vi "host.vi"() -> ()   [LabVIEW 2018]
uses:
  <vilib>/userdefined/High Color/nirio_resource_hc.ctl
  <instrlib>/niDCPower/nidcpower.llb/niDCPower Measurement Type.ctl
  <vilib>/FPGAPlugInAG/PXI-7953R/niLvFpga_Open_PXI-7953R.vi
  <vilib>/rvi/interface/common/dynamic/niFpgaDynamicAddResources.vi
  <vilib>/FPGAPlugInAG/Dynamic/niLvFpga_Reset_Dynamic.vi
  <vilib>/FPGAPlugInAG/Dynamic/niLvFpga_Run_Dynamic.vi
  <vilib>/Utility/error.llb/Error Cluster From Error Code.vi
  <vilib>/rvi/errors/niLvFpgaAdjustHostInterfaceError.vi
  <vilib>/FPGAPlugInAG/Dynamic/niLvFpga_Close_Dynamic.vi
  <vilib>/rvi/interface/nirviOpenFPGA/nirviOpenFPGA.xnode
  FPGA Bitfiles/matrix_FPGATarget_Matrixtarget_8M6uhoGy8lc.lvbitx
  <vilib>/rvi/interface/nirviMethod/nirviMethod.xnode
  <vilib>/rvi/interface/nirviReadWriteControl/nirviReadWriteControl.xnode
  <vilib>/rvi/interface/nirviCloseFPGA/nirviCloseFPGA.xnode
  <vilib>/FPGAPlugInAG/Dynamic/niLvFpga_ReadFifo_Dynamic.vi
  <vilib>/rvi/errors/niLvFpgaMergeErrorWithErrorCode.vi
  <vilib>/rvi/interface/Simulation/niFpgaSimulationCallBeginRW.vi
  <vilib>/vision/NI_Vision_Development_Module.lvlib
  NiFpgaLv.dll
panel:
  in  "57":i16=57
  in  "91":i16=91
  in  "Index - Registers Page 1":u16[](array[numeric])=[5, 6, 8, 16, 17, 18, 27, 28, 30, 37, 52, 53, 58, 59, 60, 71, 72, 76, 77, 78, 82, 83, 84, 85, 86, 87, 88, 104, 128, 129, 130, 131, 132, 133, 134, 135, 136, 137, 138, 139, 140, 141, 142, 143, 144, 145, 146, 147, 148, 149, 155, 157, 159, 160, 161, 162, 163, 164, 165, 166, 167, 168, 169, 170, 174, 175, 179, 180, 181, 182, 183, 184, 185, 186, 187, 188, 189, 190, 191, 192, 193, 194, 195, 196, 200, 220, 221, 222, 223, 224, 225, 226, 227, 240]
  in  "Registers Page 1":u16[](array[numeric])=[3, 28686, 128, 61437, 64831, 16367, 0, 0, 512, 5, 16, 61456, 512, 1066, 1024, 24, 0, 0, 0, 10, 0, 7700, 17966, 34666, 47008, 57548, 0, 17, 7, 56588, 62696, 1276, 57868, 63212, 764, 56588, 62696, 250, 34866, 56754, 63466, 2, 47646, 60627, 63473, 255, 48926, 61142, 63474, 3, 512, 9390, 0, 1280, 1280, 0, 1024, 1024, 0, 1280, 640, 0, 1024, 512, 1284, 16, 2, 32, 257, 4363, 15399, 4362, 12834, 5643, 12836, 9228, 24124, 127, 8200, 20023, 100, 8463, 19250, 100, 0, 7700, 17966, 34666, 47008, 57548, 0, 28672, 45091, 0] format="%x"
  out "Glitch Registers 2":string
  out "Glitch Registers":string
  out "glitch_num":i32
  out "Data_Read":u16=65535 format="%x"
  in  "Index - Registers Page 0":u16[](array[numeric])=[0, 1, 2, 3, 4, 5, 6, 7, 8, 9, 10, 11, 12, 13, 31, 32, 33, 34, 35, 36, 43, 44, 45, 46, 47, 48, 49, 50, 51, 52, 54, 55, 59, 60, 61, 62, 63, 64, 65, 66, 89, 90, 95, 96, 97, 98, 99, 100, 101, 112, 113, 114, 115, 116, 117, 118, 119, 120, 121, 122, 123, 124, 125, 126, 128, 129, 130, 131, 132, 133, 134, 135, 200, 240, 245, 246, 247, 248, 249, 250, 251, 252, 253, 255, 0]
  in  "Registers Page 0":u16[](array[numeric])=[5178, 12, 30, 1024, 1280, 388, 42, 190, 17, 537, 17, 0, 0, 8, 0, 768, 1036, 297, 1544, 32875, 32, 32, 32, 32, 32, 1066, 7168, 0, 841, 49177, 61680, 0, 33, 6688, 8222, 8224, 8224, 8220, 215, 1911, 12, 49167, 8989, 128, 0, 0, 0, 0, 0, 31498, 31498, 6414, 6159, 22322, 22068, 29493, 12306, 30978, 29958, 30474, 30729, 32006, 12560, 126, 127, 127, 22282, 22539, 18188, 18446, 23298, 92, 0, 0, 2047, 2047, 0, 0, 124, 0, 0, 0, 0, 5178] format="%x"
  out "number":u64=18446744073709551615 format="%b"
  in  "WRITE\nSEL_LOG":bool=TRUE caption="SEL LOGS"
  out "SEL_log file":refnum<file>
  out "IS_SEL":bool
  in  "SIM_SEL":bool
  in  "VDDIO_limit, mA":dbl=500.0 format="%#_13g"
  in  "VAA_limit, mA":dbl=500.0 format="%#_13g"
  out "selNumVAA":i32 caption="selNum"
  out "selNumVDDIO":i32 caption="selNum"
  in  "voltage level VAA":dbl=2.8 format="%#_13g"
  in  "voltage level VDD":dbl=2.8 format="%#_13g"
  in  "current limit VAA":dbl=0.10000000000000009 format="%#_13g"
  in  "current limit VDD":dbl=0.09999999999999995 format="%#_13g"
  in  "SEL":path=path "C:/VPL/LabView_PRJ/ПЕЛЕНГ_CMV4000/LOGS/SEL"
  out "Температура":string="0"
  out "Номер образца":string="0"
  out "VDDIO_Current, mA":dbl=1.2009055104110689 caption="mA" format="%_5g"
  out "VDDIO_Voltage, V":dbl=2.8003152785592405 caption="V" format="%_4g"
  out "VAA_Current, mA":dbl=14.742607861326585 caption="mA" format="%_5g"
  out "VAA_Voltage, V":dbl=2.799911738250357 caption="V" format="%_4g"
  in  "VAA - VAAPIX":refnum<k15>="PXI1Slot3"
  in  "SEL_time":u32=100
  out "Read_Low":u8=255 format="%x"
  out "Read_Up":u8=255 format="%x"
  out "TIRISTOR":bool
  in  "/RESET":bool=TRUE
  in  "DataLow":u8=231 format="%x"
  in  "Reg":u8=244 format="%x"
  in  "DataUp":u8=2 format="%x"
  in  "Device":u8=186 format="%x"
  in  "VDD_limit, mA":dbl=500.0 format="%#_13g"
  out "selNumVDD":i32 caption="selNum"
  out "Ready":bool=TRUE
  in  "output enabled":bool=TRUE
  out "VDD_Current, mA":dbl=-0.2678676595787411 caption="mA" format="%_5g"
  out "VDD_Voltage, V":dbl=2.801952990328096 caption="V" format="%_4g"
  in  "VDDIO - VDD":refnum<k15>="PXI1Slot2"
  in  "Comand":T1(ring)=enum."From Controls"
  in  "Height_pix":i32=250
  in  "Width_pix":i32=250
  in  "55":i16=55
  in  "73":i16=73
  in  "75":i16=75
  in  "56":i16=56
  in  "55":i16=55
  in  "Comand":bool
  out "ACK":u8 format="%b"
  out "String_counter":i16=250
  in  "String_number":i16=250
  in  "I2C_Request":bool
  in  "FALSE_LV":bool
  in  "FALSE_PIXCLK":bool=TRUE
  in  "TRUE_FV":bool=TRUE
  in  "1_EXTCLK_divider":i16=5
  out "Image":T2(plugin-control)
  in  "0_WE divider":i32
  in  "50_Rise/Fall divider":i32=50
  in  "72":i16=72
  in  "18":i16=18
  in  "36":i16=36
  in  "54":i16=54
  in  "71":i16=71
  in  "17":i16=17
  in  "35":i16=35
  in  "53":i16=53
  in  "75_Stop":i16=75
  in  "100_Sclk_divider":i32=100
  in  "Read1":u8=255 format="%x"
  in  "Read2":u8=255 format="%x"
  in  "I2C_Write":bool
  in  "stop":bool=TRUE
  out "ArrayUp":u64=1534
  out "ArrayLow":u64=2298524764643157990
  in  "resource name":T3="PXI1Slot6" caption="RIO Device"
  out "Сколько вначале":u32=262142
  out "Data":u8[](array[numeric])
  # "YCbCr mode"
  # "VDD"
  # "VDDIO"
  # "VAA"
  # "RGB565"
  # "I2C"
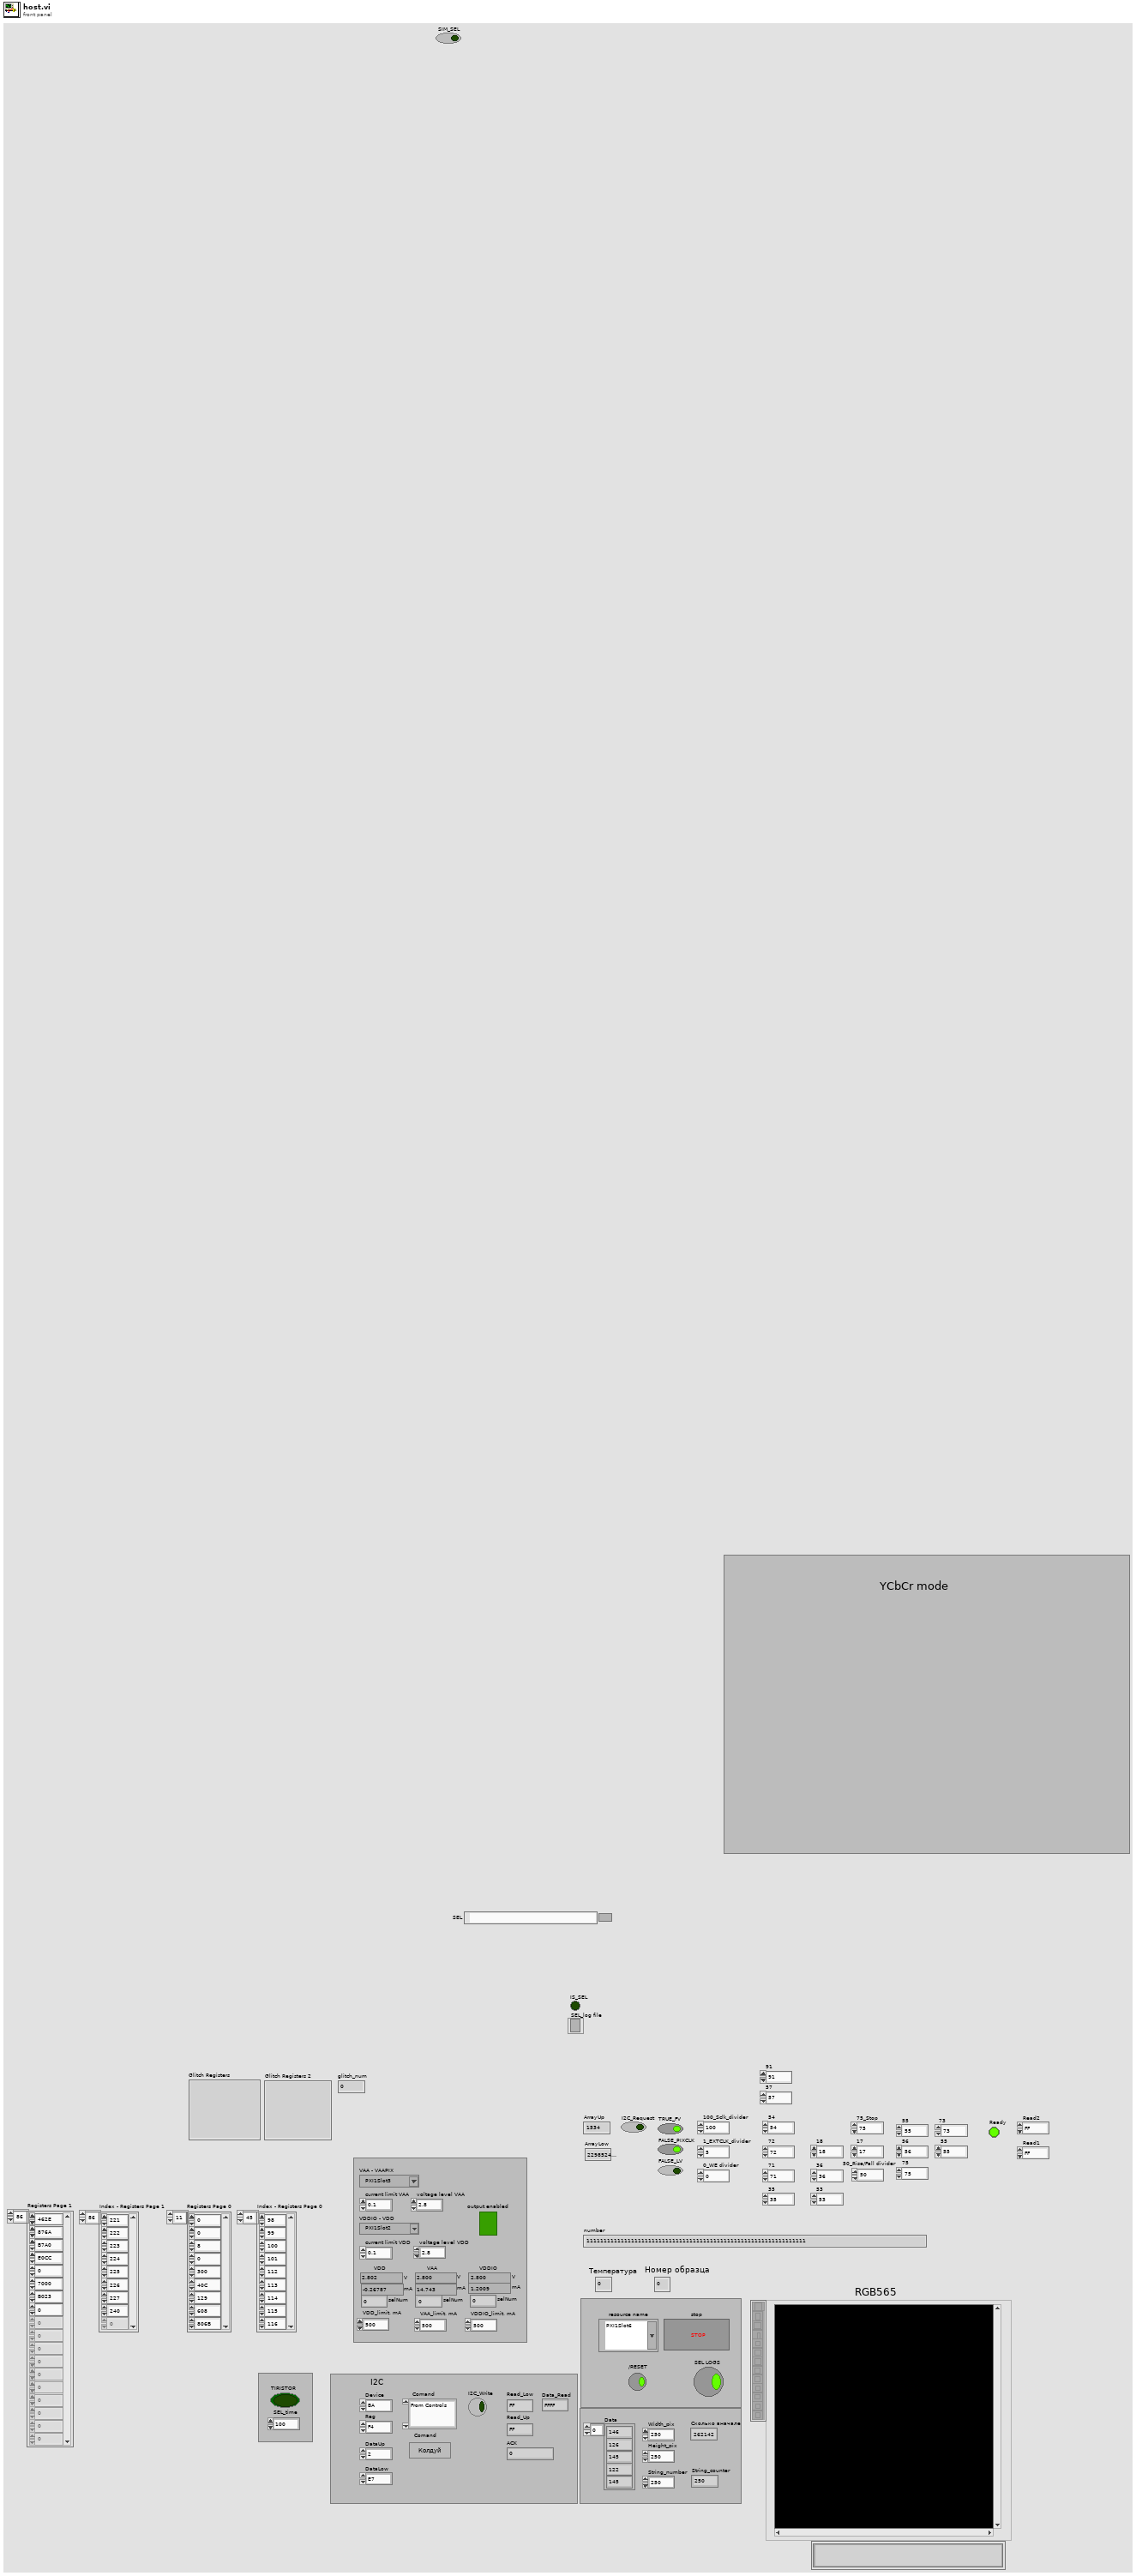
[diagram p1: front panel]
types:
  T1 = enum16{"check_registers", "From Controls", "250x250", "RGB565"}
  T2 = typedef "IMAQ Image.ctl" = refnum<image>
  T3 = typedef "nirio_resource_hc.ctl" = tag
  T4 = enum16{"open", "replace", "create", "open or create", "replace or create", "replace or create with confirmation"}
  T5 = typedef "Image Type" = u32
  T6 = typedef "niDCPower Measurement Type.ctl" = i32
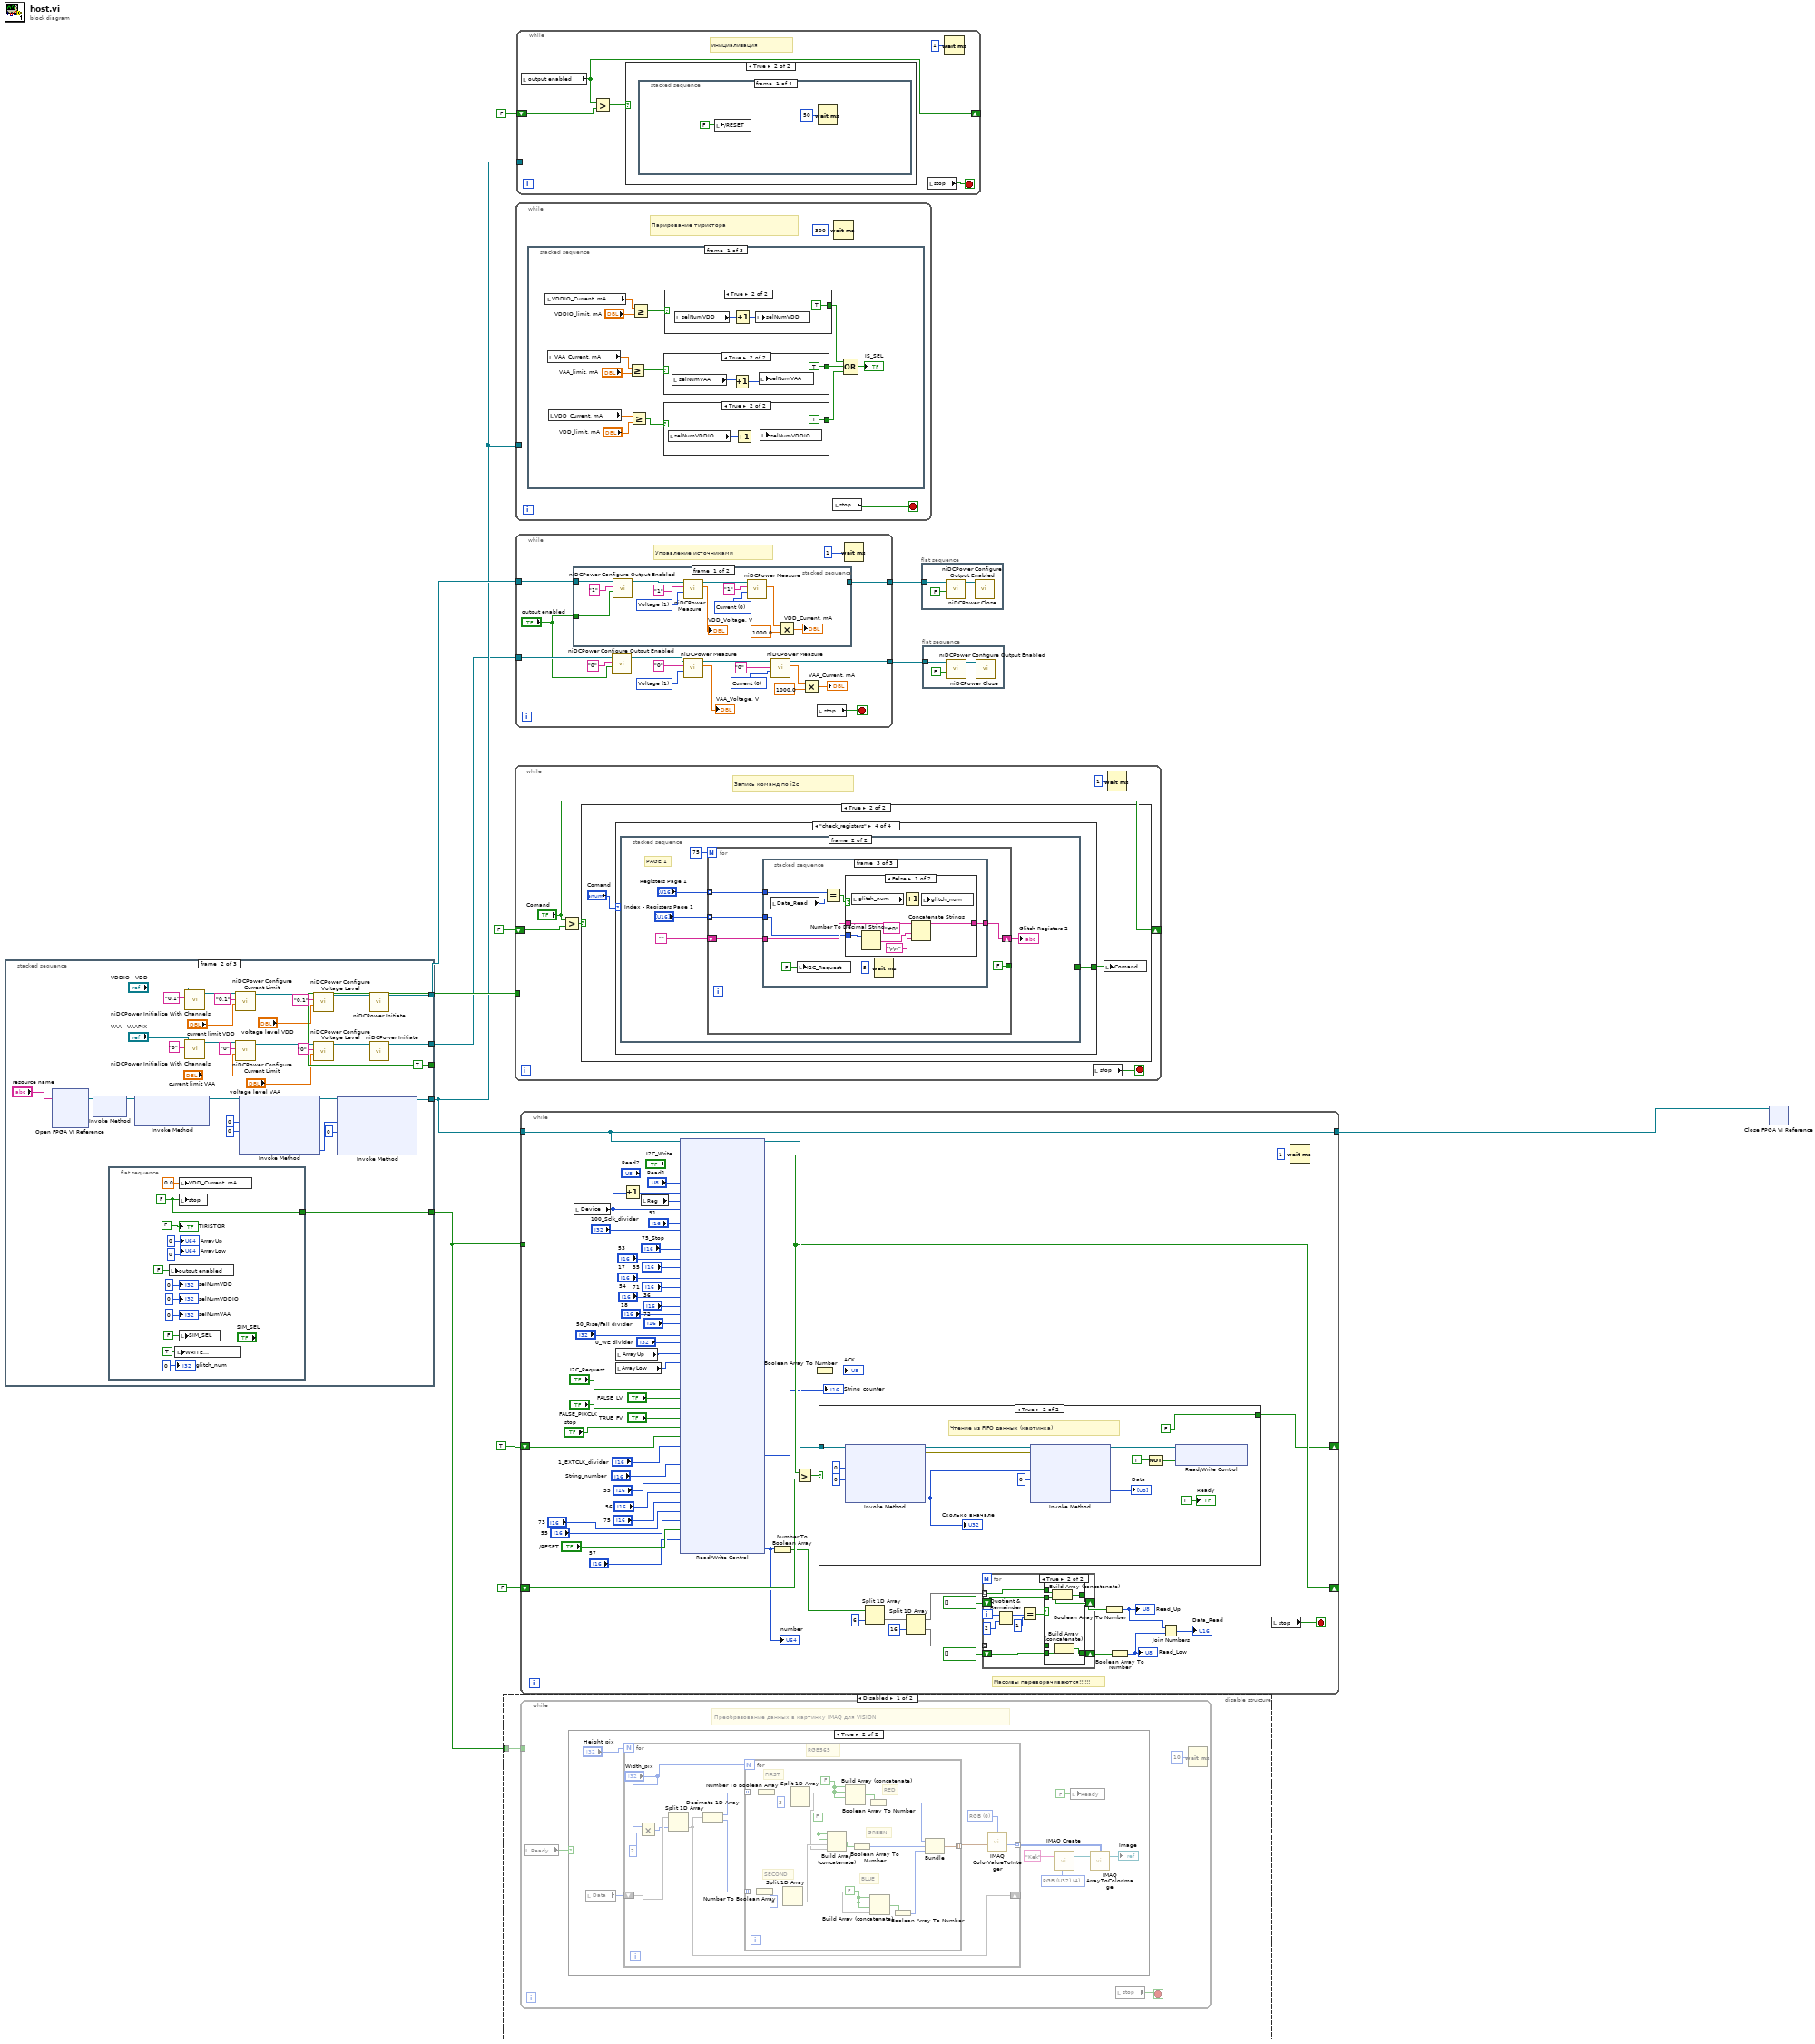
[diagram p0: block diagram]
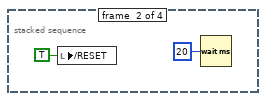
[diagram p5: hidden frame]
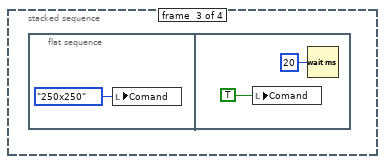
[diagram p6: hidden frame]
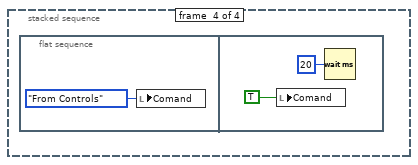
[diagram p7: hidden frame]
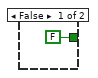
[diagram p8: hidden frame]
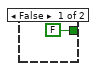
[diagram p9: hidden frame]
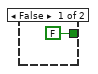
[diagram p10: hidden frame]
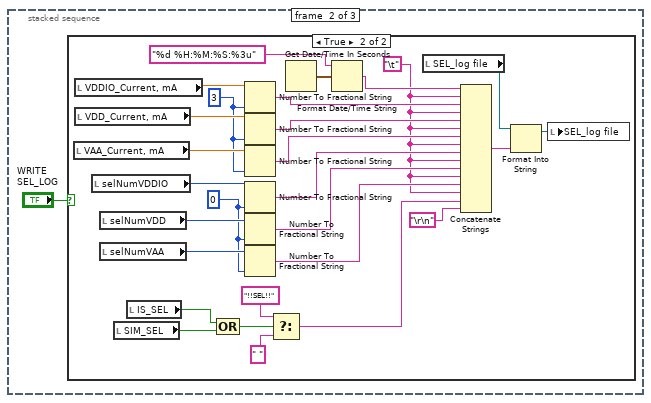
[diagram p11: hidden frame]
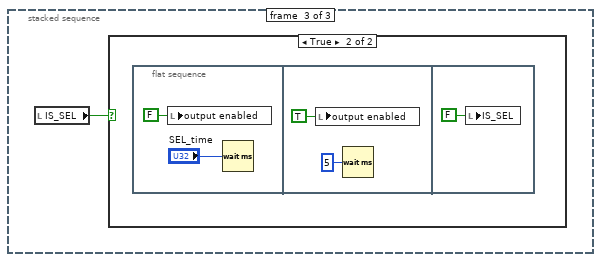
[diagram p13: hidden frame]
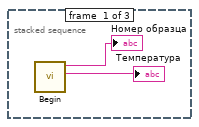
[diagram p15: hidden frame]
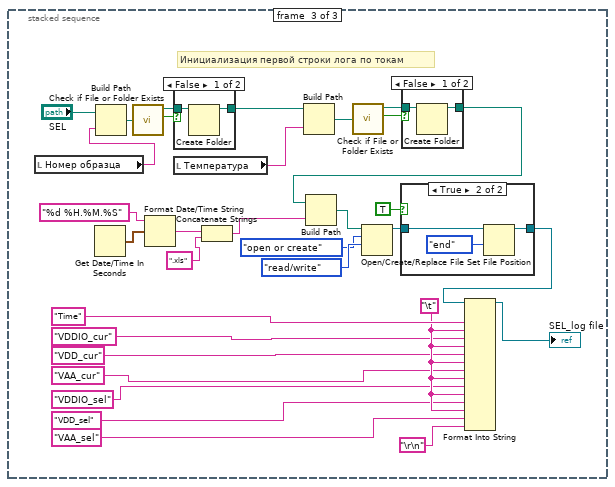
[diagram p16: hidden frame]
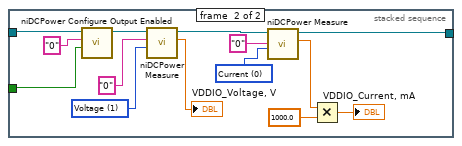
[diagram p20: hidden frame]
diagram:
  n1 = stacked-sequence {
    tunnel: [_ w46 _] -> w3
    tunnel: [_ w27 _] -> w5
    tunnel: [_ w26 _] -> w7
    tunnel: [_ TRUE _] -> w6
    tunnel: [_ w15 _] -> w2
    frame #0 {
      n2 = call "Begin.vi"() -> ("Температура 2"=→"Температура":string, "Номер образца 2"=→"Номер образца":string)  [unwired: 10 in]
    }
    frame #1 {
      n3 = xnode "Open FPGA VI Reference"("resource name"="resource name") -> ("FPGA VI Reference Out"=w36:refnum<k20>)  [unwired: 1 in, 1 out]
      n4 = xnode "Invoke Method"("FPGA VI Reference In"=w36) -> ("FPGA VI Reference Out"=w35:refnum<k20>)  [unwired: 1 in, 1 out]
      n5 = flat-sequence {
        tunnel: [w58] -> w27
        frame #0 {
          w58 = FALSE ("СТОП ПЛИС")
          n6 = local write "output enabled"(FALSE ("output enabled")) -> ()
          n7 = local write "WRITE\nSEL_LOG"(TRUE ("WRITE\nSEL_LOG")) -> ()
          n8 = local write "VDD_Current, mA"(0.0 ("Ch1_Current, mA")) -> ()
          n9 = local write "stop"(w58) -> ()
          n10 = local write "SIM_SEL"(FALSE ("SIM_SEL")) -> ()
          "ArrayLow" <- u64 0 ("ArrayLow")
          "ArrayUp" <- u64 0 ("ArrayUp")
          "selNumVDD" <- 0 ("Numeric")
          "TIRISTOR" <- FALSE ("TIRISTOR")
          "selNumVDDIO" <- 0 ("Numeric")
          "selNumVAA" <- 0 ("Numeric")
          "glitch_num" <- 0 ("glitch_num")
        }
      }
      n11 = xnode "Invoke Method"("FPGA VI Reference In"=w35) -> ("FPGA VI Reference Out"=w33:refnum<k20>)  [unwired: 2 in, 1 out]
      n12 = call <instrlib>:"niDCPower Initialize With Channels.vi"("channels"="0,1", "resource name"="VDDIO - VDD") -> ("instrument handle out"=w37:refnum<k15>)  [unwired: 8 in, 1 out]
      n13 = call <instrlib>:"niDCPower Initialize With Channels.vi"("channels"="0", "resource name"="VAA - VAAPIX") -> ("instrument handle out"=w16:refnum<k15>)  [unwired: 8 in, 1 out]
      n14 = call <instrlib>:"niDCPower Configure Current Limit.vi"("current limit"="current limit VDD", "channel name"="0,1", "instrument handle"=w37) -> ("instrument handle out"=w38:refnum<k15>)  [unwired: 7 in, 1 out]
      n15 = call <instrlib>:"niDCPower Configure Current Limit.vi"("current limit"="current limit VAA", "channel name"="0", "instrument handle"=w16) -> ("instrument handle out"=w17:refnum<k15>)  [unwired: 7 in, 1 out]
      n16 = xnode "Invoke Method"("FPGA VI Reference In"=w33, "Number of Elements"=u32 0, "Timeout (ms)"=0) -> ("FPGA VI Reference Out"=w31:refnum<k20>, "Elements Remaining"=w32:u32)  [unwired: 1 in, 2 out]
      n17 = call <instrlib>:"niDCPower Configure Voltage Level.vi"("voltage level"="voltage level VDD", "channel name"="0,1", "instrument handle"=w38) -> ("instrument handle out"=w39:refnum<k15>)  [unwired: 7 in, 1 out]
      n18 = call <instrlib>:"niDCPower Configure Voltage Level.vi"("voltage level"="voltage level VAA", "channel name"="0", "instrument handle"=w17) -> ("instrument handle out"=w18:refnum<k15>)  [unwired: 7 in, 1 out]
      n19 = xnode "Invoke Method"("FPGA VI Reference In"=w31, "Number of Elements"=w32, "Timeout (ms)"=0) -> ("FPGA VI Reference Out"=w46:refnum<k20>)  [unwired: 1 in, 3 out]
      n20 = call <instrlib>:"niDCPower Initiate.vi"("instrument handle"=w39) -> ("instrument handle out"=w26:refnum<k15>)  [unwired: 9 in, 1 out]
      n21 = call <instrlib>:"niDCPower Initiate.vi"("instrument handle"=w18) -> ("instrument handle out"=w15:refnum<k15>)  [unwired: 9 in, 1 out]
    }
    frame #2 {
      w67 = "\t"
      # "Инициализация первой строки лога по токам"
      n22 = local read "Номер образца"() -> (w78:string)
      n23 = Get Date/Time In Seconds() -> (seconds since 1Jan1904=w83:timestamp)
      n24 = Build Path(base path="SEL", name or relative path=w78) -> (appended path=w76:path)
      n25 = call <vilib>:"Check if File or Folder Exists.vi"("path"=w76) -> ("file or folder exists?"=w75:bool, "dup path"=w74:path)  [unwired: 8 in, 1 out]
      n26 = Format Date/Time String(time format string (%c)="%d %H.%M.%S", seconds (now)=w83) -> (date/time string=w85:string)  [unwired: 1 in]
      n27 = case shown="False" w75 {
        tunnel: w74 -> [w99 w100]
        tunnel: [w98 w100] -> w80
        frame False {
          n28 = Create Folder(path (use dialog)=w99) -> (created path=w98:path)  [unwired: 2 in, 2 out]
        }
        frame True {
        }
      }
      n29 = local read "Температура"() -> (w81:string)
      n30 = Concatenate Strings(w85, ".xls" ("string")) -> (w86:string)
      n31 = Build Path(base path=w80, name or relative path=w81) -> (appended path=w89:path)
      n32 = call <vilib>:"Check if File or Folder Exists.vi"("path"=w89) -> ("file or folder exists?"=w90:bool, "dup path"=w79:path)  [unwired: 8 in, 1 out]
      n33 = case shown="False" w90 {
        tunnel: w79 -> [w96 w97]
        tunnel: [w95 w97] -> w87
        frame False {
          n34 = Create Folder(path (use dialog)=w96) -> (created path=w95:path)  [unwired: 2 in, 2 out]
        }
        frame True {
        }
      }
      n35 = Build Path(base path=w87, name or relative path=w86) -> (appended path=w84:path)
      n36 = Open/Create/Replace File(file path (use dialog)=w84, operation (0:open)=T4."open or create", access (0:read/write)=enum16{"read/write", "read-only", "write-only"}."read/write") -> (refnum out=w82:refnum<file>)  [unwired: 3 in, 2 out]
      n37 = case shown="True" TRUE {
        tunnel: w82 -> [w91 w94]
        tunnel: [w91 w92] -> w88
        frame False {
        }
        frame True {
          n38 = Set File Position(refnum=w94, from (0:start)=enum16{"start", "end", "current"}."end") -> (refnum out=w92:refnum<file>)  [unwired: 2 in, 1 out]
        }
      }
      n39 = Format Into String(initial string=w88, "Time" ("input 1"), w67, "VDDIO_cur" ("input 1"), w67, "VDD_cur" ("input 1"), w67, "VAA_cur" ("input 1"), w67, "VDDIO_sel" ("input 1"), w67, "VDD_sel" ("input 1"), w67, "VAA_sel" ("input 1"), "\r\n") -> (resulting string=→"SEL_log file":refnum<file>)  [unwired: 2 in, 1 out]
    }
  }
  n40 = disable-structure shown="Disabled" {
    disable-tunnel: w5 -> [w101 _]
    frame Disabled {
      n41 = while {
        tunnel: w101 -> [_]
        stop <- w104 stop-if-true
        # "Преобразование данных в картинку IMAQ для VISION"
        n42 = local read "Ready"() -> (w102:bool)
        n43 = case shown="True" w102 {
          frame False {
          }
          frame True {
            w111 = T5 4 items=["Grayscale (U8)", "Grayscale (I16)", "Grayscale (SGL)", "Complex (CSG)", "RGB (U32)", "HSL (U32)", "RGB (U64)"] ("Image Type")
            n44 = local read "Data"() -> (w106:u8[])
            n45 = for {
              N: "Height_pix" -> [_]
              shift-right: [w118] -> _
              shift-left: w106 -> [w115]
              tunnel: [w116] -> w107 mode=indexing
              w120 = u16 0 items=["RGB", "HSL", "HSV", "HSI"] ("Color Mode")
              # "RGB565"
              n46 = Multiply(x="Width_pix", y=2) -> (x*y=w114:i32)
              n47 = Split 1D Array(array=w115, index=w114) -> (second subarray=w118:u8[])  [unwired: 1 out]
              n48 = Decimate 1D Array(w118) -> (w122:u8[], w121:u8[])
              n49 = for {
                N: "Width_pix" -> [_]
                tunnel: w122 -> [w141] mode=indexing
                tunnel: w121 -> [w142] mode=indexing
                tunnel: [w123] -> w117 mode=indexing
                w131 = FALSE
                w132 = FALSE
                w133 = FALSE
                # "BLUE"
                # "GREEN"
                # "RED"
                # "SECOND"
                # "FIRST"
                n50 = Number To Boolean Array(number=w142) -> (Boolean array=w137:bool[])
                n51 = Number To Boolean Array(number=w141) -> (Boolean array=w140:bool[])
                n52 = Split 1D Array(array=w137, index=5) -> (first subarray=w129:bool[], second subarray=w136:bool[])
                n53 = Split 1D Array(array=w140, index=3) -> (first subarray=w128:bool[], second subarray=w127:bool[])
                n54 = Build Array (concatenate)(w132, w132, w136, w128) -> (w135:bool[])
                n55 = Build Array (concatenate)(w133, w133, w133, w127) -> (w134:bool[])
                n56 = Boolean Array To Number(Boolean array=w135) -> (number=w125:u8)
                n57 = Boolean Array To Number(Boolean array=w134) -> (number=w124:u8)
                n58 = Build Array (concatenate)(w131, w131, w131, w129) -> (w130:bool[])
                n59 = Boolean Array To Number(Boolean array=w130) -> (number=w126:u8)
                n60 = Bundle(w124, w125, w126) -> (w123:cluster{u8, u8, u8})  [unwired: 1 in]
              }
              n61 = call "IMAQ ColorValueToInteger"("1D Color value array"=w117, "Color Mode"=w120) -> ("1D U32 array"=w116:u32[])  [unwired: 3 in, 3 out]
            }
            n62 = call "IMAQ Create"("Image Name"="Kek", "Image Type"=w111) -> ("New Image"=w110:T2)  [unwired: 3 in, 1 out]
            n63 = local write "Ready"(FALSE ("Ready")) -> ()
            n64 = call "IMAQ ArrayToColorImage"("Image Pixels (U32)"=w107, "Image"=w110) -> ("Image Out"=→"Image":T2)  [unwired: 3 in, 1 out]
          }
        }
        n65 = local read "stop"() -> (w104:bool)
        n66 = Wait (ms)(milliseconds to wait=u32 10) -> ()  [unwired: 1 out]
      }
    }
    frame Enabled {
    }
  }
  n67 = while {
    shift-right: ["Comand"] -> _
    shift-left: FALSE -> [w145]
    tunnel: w6 -> [_]
    stop <- w147 stop-if-true
    # "Запись команд по i2c"
    n68 = Greater?(x="Comand", y=w145) -> (0:w146:bool)
    n69 = case shown="True" w146 {
      frame False {
      }
      frame True {
        n70 = case shown="\"check_registers\"" "Comand" {
          tunnel: [w150 w176 w201 w213] -> w148
          frame "RGB565" {
            n71 = stacked-sequence {
              tunnel: [_ w162] -> w150
              frame #0 {
                n72 = flat-sequence {
                  frame #0 {
                    n73 = local write "I2C_Write"(TRUE ("I2C_Write")) -> ()
                    n74 = call "I2C_Write.vi"("DataLow"=u8 1 ("Device"), "DataUp"=u8 0 ("Device"), "Reg"=u8 240 ("Device"), "Device"=u8 186) -> ("ArrayLow"=w156:u64, "ArrayUp"=w155:u64)  [unwired: 6 in]
                    n75 = local write "ArrayUp"(w155) -> ()
                    n76 = local write "ArrayLow"(w156) -> ()
                  }
                  frame #1 {
                    n77 = local write "I2C_Request"(TRUE ("I2C_Request")) -> ()
                    n78 = Wait (ms)(milliseconds to wait=u32 5) -> ()  [unwired: 1 out]
                  }
                  frame #2 {
                    n79 = local write "I2C_Request"(FALSE ("I2C_Request")) -> ()
                    n80 = Wait (ms)(milliseconds to wait=u32 5) -> ()  [unwired: 1 out]
                  }
                }
              }
              frame #1 {
                n81 = flat-sequence {
                  tunnel: [FALSE ("RGB565")] -> w162
                  frame #0 {
                    n82 = local write "I2C_Write"(TRUE ("I2C_Write")) -> ()
                    n83 = call "I2C_Write.vi"("DataLow"=u8 0 ("Device"), "DataUp"=u8 3 ("Device"), "Reg"=u8 58 ("Device"), "Device"=u8 186) -> ("ArrayLow"=w168:u64, "ArrayUp"=w167:u64)  [unwired: 6 in]
                    n84 = local write "ArrayUp"(w167) -> ()
                    n85 = local write "ArrayLow"(w168) -> ()
                  }
                  frame #1 {
                    n86 = local write "I2C_Request"(TRUE ("I2C_Request")) -> ()
                    n87 = Wait (ms)(milliseconds to wait=u32 2) -> ()  [unwired: 1 out]
                  }
                  frame #2 {
                    n88 = local write "I2C_Request"(FALSE ("I2C_Request")) -> ()
                    n89 = Wait (ms)(milliseconds to wait=u32 2) -> ()  [unwired: 1 out]
                  }
                }
              }
            }
          }
          frame "250x250" {
            w175 = 250 ("Height_pix")
            n90 = stacked-sequence {
              tunnel: [_ w188] -> w176
              frame #0 {
                n91 = flat-sequence {
                  frame #0 {
                    n92 = local write "I2C_Write"(TRUE ("I2C_Write")) -> ()
                    n93 = call "I2C_Write.vi"("DataLow"=u8 0 ("Device"), "DataUp"=u8 0 ("Device"), "Reg"=u8 240 ("Device"), "Device"=u8 186) -> ("ArrayLow"=w182:u64, "ArrayUp"=w181:u64)  [unwired: 6 in]
                    n94 = local write "ArrayUp"(w181) -> ()
                    n95 = local write "ArrayLow"(w182) -> ()
                  }
                  frame #1 {
                    n96 = local write "I2C_Request"(TRUE ("I2C_Request")) -> ()
                    n97 = Wait (ms)(milliseconds to wait=u32 10) -> ()  [unwired: 1 out]
                  }
                  frame #2 {
                    n98 = local write "I2C_Request"(FALSE ("I2C_Request")) -> ()
                    n99 = Wait (ms)(milliseconds to wait=u32 10) -> ()  [unwired: 1 out]
                  }
                }
              }
              frame #1 {
                n100 = flat-sequence {
                  tunnel: [FALSE ("RGB565")] -> w188
                  frame #0 {
                    n101 = local write "I2C_Write"(TRUE ("I2C_Write")) -> ()
                    n102 = call "I2C_Write.vi"("DataLow"=u8 231 ("Device"), "DataUp"=u8 1 ("Device"), "Reg"=u8 4 ("Device"), "Device"=u8 186) -> ("ArrayLow"=w190:u64, "ArrayUp"=w189:u64)  [unwired: 6 in]
                    n103 = local write "ArrayUp"(w189) -> ()
                    n104 = local write "ArrayLow"(w190) -> ()
                  }
                  frame #1 {
                    n105 = local write "I2C_Request"(TRUE ("I2C_Request")) -> ()
                    n106 = Wait (ms)(milliseconds to wait=u32 10) -> ()  [unwired: 1 out]
                  }
                  frame #2 {
                    n107 = local write "I2C_Request"(FALSE ("I2C_Request")) -> ()
                    n108 = Wait (ms)(milliseconds to wait=u32 10) -> ()  [unwired: 1 out]
                  }
                }
              }
            }
            n109 = local write "String_number"(w175) -> ()
            n110 = local write "Width_pix"(w175) -> ()
            n111 = local write "Height_pix"(w175) -> ()
          }
          frame "From Controls" {
            n112 = flat-sequence {
              tunnel: [FALSE] -> w201
              frame #0 {
                n113 = call "I2C_Write.vi"("DataLow"="DataLow", "DataUp"="DataUp", "Reg"="Reg", "Device"="Device") -> ("ArrayLow"=w203:u64, "ArrayUp"=w202:u64)  [unwired: 6 in]
                n114 = local write "ArrayUp"(w202) -> ()
                n115 = local write "ArrayLow"(w203) -> ()
              }
              frame #1 {
                n116 = local write "I2C_Request"(TRUE ("I2C_Request")) -> ()
                n117 = Wait (ms)(milliseconds to wait=u32 5) -> ()  [unwired: 1 out]
              }
              frame #2 {
                n118 = local write "I2C_Request"(FALSE ("I2C_Request")) -> ()
                n119 = Wait (ms)(milliseconds to wait=u32 5) -> ()  [unwired: 1 out]
              }
            }
          }
          frame "check_registers" {
            n120 = stacked-sequence {
              tunnel: [w215 _] -> w213
              frame #0 {
                # "PAGE 0"
                n121 = for {
                  N: 82 -> [_]
                  tunnel: "Index - Registers Page 0" -> [w224] mode=indexing
                  tunnel: "Registers Page 0" -> [w223] mode=indexing
                  shift-right: [w221] -> w216
                  shift-left: "" -> [w222]
                  tunnel: [FALSE] -> w215
                  n122 = stacked-sequence {
                    tunnel: w224 -> [w225 _ w229]
                    tunnel: w223 -> [_ _ w233]
                    tunnel: w222 -> [_ _ w231]
                    tunnel: [_ _ w230] -> w221
                    frame #0 {
                      n123 = local write "Device"(u8 186 ("Device")) -> ()
                      n124 = local write "Reg"(w225) -> ()
                    }
                    frame #1 {
                      n125 = local write "I2C_Request"(TRUE ("I2C_Request")) -> ()
                      n126 = Wait (ms)(milliseconds to wait=u32 5) -> ()  [unwired: 1 out]
                    }
                    frame #2 {
                      n127 = local read "Data_Read"() -> (w234:u16)
                      n128 = local write "I2C_Request"(FALSE ("I2C_Request")) -> ()
                      n129 = Equal?(x=w233, y=w234) -> (x = y?=w232:bool)
                      n130 = case shown="False" w232 {
                        tunnel: w231 -> [w242 w245]
                        tunnel: [w241 w245] -> w230
                        tunnel: w229 -> [w239 _]
                        frame False {
                          n131 = local read "glitch_num"() -> (w244:i32)
                          n132 = Number To Decimal String(number=w239) -> (decimal integer string=w238:string)  [unwired: 1 in]
                          n133 = Increment(x=w244) -> (x+1=w243:i32)
                          n134 = Concatenate Strings(w242, "#R" ("string"), w238, "\r\n") -> (w241:string)
                          n135 = local write "glitch_num"(w243) -> ()
                        }
                        frame True {
                        }
                      }
                      n136 = Wait (ms)(milliseconds to wait=u32 5) -> ()  [unwired: 1 out]
                    }
                  }
                }
                "Glitch Registers" <- w216
              }
              frame #1 {
                # "PAGE 1"
                n137 = for {
                  N: 75 -> [_]
                  tunnel: "Index - Registers Page 1" -> [w255] mode=indexing
                  tunnel: "Registers Page 1" -> [w254] mode=indexing
                  shift-right: [w252] -> w248
                  shift-left: "" -> [w253]
                  tunnel: [FALSE] -> _
                  n138 = stacked-sequence {
                    tunnel: w255 -> [w256 _ w260]
                    tunnel: w254 -> [_ _ w264]
                    tunnel: w253 -> [_ _ w262]
                    tunnel: [_ _ w261] -> w252
                    frame #0 {
                      n139 = local write "Device"(u8 186 ("Device")) -> ()
                      n140 = local write "Reg"(w256) -> ()
                    }
                    frame #1 {
                      n141 = local write "I2C_Request"(TRUE ("I2C_Request")) -> ()
                      n142 = Wait (ms)(milliseconds to wait=u32 5) -> ()  [unwired: 1 out]
                    }
                    frame #2 {
                      n143 = local read "Data_Read"() -> (w265:u16)
                      n144 = local write "I2C_Request"(FALSE ("I2C_Request")) -> ()
                      n145 = Equal?(x=w264, y=w265) -> (x = y?=w263:bool)
                      n146 = case shown="False" w263 {
                        tunnel: w262 -> [w273 w276]
                        tunnel: [w272 w276] -> w261
                        tunnel: w260 -> [w270 _]
                        frame False {
                          n147 = local read "glitch_num"() -> (w275:i32)
                          n148 = Number To Decimal String(number=w270) -> (decimal integer string=w269:string)  [unwired: 1 in]
                          n149 = Increment(x=w275) -> (x+1=w274:i32)
                          n150 = Concatenate Strings(w273, "#R" ("string"), w269, "\r\n") -> (w272:string)
                          n151 = local write "glitch_num"(w274) -> ()
                        }
                        frame True {
                        }
                      }
                      n152 = Wait (ms)(milliseconds to wait=u32 5) -> ()  [unwired: 1 out]
                    }
                  }
                }
                "Glitch Registers 2" <- w248
              }
            }
          }
        }
        n153 = local write "Comand"(w148) -> ()
      }
    }
    n154 = local read "stop"() -> (w147:bool)
    n155 = Wait (ms)(milliseconds to wait=u32 1) -> ()  [unwired: 1 out]
  }
  n156 = while {
    tunnel: w3 -> [_]
    stop <- w278 stop-if-true
    # "Парирование тиристора"
    n157 = stacked-sequence {
      frame #0 {
        n158 = local read "VDDIO_Current, mA"() -> (w286:dbl)
        n159 = local read "VAA_Current, mA"() -> (w287:dbl)
        n160 = local read "VDD_Current, mA"() -> (w291:dbl)
        n161 = Greater Or Equal?(x=w287, y="VAA_limit, mA") -> (x >= y?=w283:bool)
        n162 = Greater Or Equal?(x=w291, y="VDD_limit, mA") -> (x >= y?=w281:bool)
        n163 = Greater Or Equal?(x=w286, y="VDDIO_limit, mA") -> (x >= y?=w285:bool)
        n164 = case shown="True" w283 {
          tunnel: [FALSE TRUE] -> w282
          frame False {
          }
          frame True {
            n165 = local read "selNumVAA"() -> (w299:i32)
            n166 = Increment(x=w299) -> (x+1=w298:i32)
            n167 = local write "selNumVAA"(w298) -> ()
          }
        }
        n168 = case shown="True" w281 {
          tunnel: [FALSE TRUE] -> w280
          frame False {
          }
          frame True {
            n169 = local read "selNumVDDIO"() -> (w295:i32)
            n170 = Increment(x=w295) -> (x+1=w294:i32)
            n171 = local write "selNumVDDIO"(w294) -> ()
          }
        }
        n172 = case shown="True" w285 {
          tunnel: [FALSE TRUE] -> w284
          frame False {
          }
          frame True {
            n173 = local read "selNumVDD"() -> (w303:i32)
            n174 = Increment(x=w303) -> (x+1=w302:i32)
            n175 = local write "selNumVDD"(w302) -> ()
          }
        }
        n176 = Compound Arithmetic op=OR(w284, w282, w280) -> (→"IS_SEL":bool)
      }
      frame #1 {
        n177 = case shown="True" "WRITE\nSEL_LOG" {
          frame False {
          }
          frame True {
            w311 = i16 0 ("width (-)")
            w310 = i16 3 ("width (-)")
            w308 = "\t"
            n178 = local read "VAA_Current, mA"() -> (w325:dbl)
            n179 = local read "VDDIO_Current, mA"() -> (w323:dbl)
            n180 = local read "VDD_Current, mA"() -> (w324:dbl)
            n181 = local read "selNumVDDIO"() -> (w326:i32)
            n182 = local read "selNumVDD"() -> (w327:i32)
            n183 = local read "selNumVAA"() -> (w328:i32)
            n184 = local read "SIM_SEL"() -> (w315:bool)
            n185 = local read "IS_SEL"() -> (w316:bool)
            n186 = Compound Arithmetic op=OR(w316, w315) -> (w332:bool)
            n187 = Number To Fractional String(number=w323, precision (6)=w310) -> (F-format string=w329:string)  [unwired: 2 in]
            n188 = Number To Fractional String(number=w324, precision (6)=w310) -> (F-format string=w330:string)  [unwired: 2 in]
            n189 = Number To Fractional String(number=w325, precision (6)=w310) -> (F-format string=w331:string)  [unwired: 2 in]
            n190 = Number To Fractional String(number=w326, precision (6)=w311) -> (F-format string=w319:string)  [unwired: 2 in]
            n191 = Number To Fractional String(number=w327, precision (6)=w311) -> (F-format string=w318:string)  [unwired: 2 in]
            n192 = Number To Fractional String(number=w328, precision (6)=w311) -> (F-format string=w317:string)  [unwired: 2 in]
            n193 = Select(t="!!SEL!!", s=w332, f=" ") -> (s? t:f=w314:string)
            n194 = Get Date/Time In Seconds() -> (seconds since 1Jan1904=w320:timestamp)
            n195 = Format Date/Time String(time format string (%c)="%d %H:%M:%S:%3u", seconds (now)=w320) -> (date/time string=w322:string)  [unwired: 1 in]
            n196 = local read "SEL_log file"() -> (w306:refnum<file>)
            n197 = Concatenate Strings(w322, w308, w329, w308, w330, w308, w331, w308, w319, w308, w318, w308, w317, w308, w314, "\r\n") -> (w321:string)
            n198 = Format Into String(initial string=w306, w321) -> (resulting string=w305:refnum<file>)  [unwired: 2 in, 1 out]
            n199 = local write "SEL_log file"(w305) -> ()
          }
        }
      }
      frame #2 {
        n200 = local read "IS_SEL"() -> (w333:bool)
        n201 = case shown="True" w333 {
          frame False {
          }
          frame True {
            n202 = flat-sequence {
              frame #0 {
                n203 = local write "output enabled"(FALSE ("output enabled")) -> ()
                n204 = Wait (ms)(milliseconds to wait="SEL_time") -> ()  [unwired: 1 out]
              }
              frame #1 {
                n205 = local write "output enabled"(TRUE ("output enabled")) -> ()
                n206 = Wait (ms)(milliseconds to wait=u32 5) -> ()  [unwired: 1 out]
              }
              frame #2 {
                n207 = local write "IS_SEL"(FALSE ("IS_SEL")) -> ()
              }
            }
          }
        }
      }
    }
    n208 = local read "stop"() -> (w278:bool)
    n209 = Wait (ms)(milliseconds to wait=u32 300) -> ()  [unwired: 1 out]
  }
  n210 = while {
    tunnel: w7 -> [w355]
    tunnel: [w354] -> w9
    tunnel: w2 -> [w341]
    tunnel: [w342] -> w1
    stop <- w356 stop-if-true
    w345 = T6 0 items=["Current", "Voltage"] ("measurement type")
    w346 = T6 1 items=["Current", "Voltage"] ("measurement type")
    # "Управление источниками"
    n211 = stacked-sequence {
      tunnel: w355 -> [w367 w372]
      tunnel: [_ w371] -> w354
      tunnel: "output enabled" -> [w357 w373]
      frame #0 {
        w360 = T6 0 items=["Current", "Voltage"] ("measurement type")
        w361 = T6 1 items=["Current", "Voltage"] ("measurement type")
        n212 = call <instrlib>:"niDCPower Configure Output Enabled.vi"("output enabled"=w357, "channel name"="1", "instrument handle"=w367) -> ("instrument handle out"=w369:refnum<k15>)  [unwired: 7 in, 1 out]
        n213 = call <instrlib>:"niDCPower Measure.vi"("measurement type"=w361, "channel name"="1", "instrument handle"=w369) -> ("measurement"=→"VDD_Voltage, V":dbl, "instrument handle out"=w366:refnum<k15>)  [unwired: 6 in, 1 out]
        n214 = call <instrlib>:"niDCPower Measure.vi"("measurement type"=w360, "channel name"="1", "instrument handle"=w366) -> ("measurement"=w362:dbl)  [unwired: 6 in, 2 out]
        n215 = Multiply(x=w362, y=1000.0) -> (x*y=→"VDD_Current, mA":dbl)
      }
      frame #1 {
        w378 = T6 0 items=["Current", "Voltage"] ("measurement type")
        w376 = T6 1 items=["Current", "Voltage"] ("measurement type")
        n216 = call <instrlib>:"niDCPower Configure Output Enabled.vi"("output enabled"=w373, "channel name"="0", "instrument handle"=w372) -> ("instrument handle out"=w380:refnum<k15>)  [unwired: 7 in, 1 out]
        n217 = call <instrlib>:"niDCPower Measure.vi"("measurement type"=w376, "channel name"="0", "instrument handle"=w380) -> ("measurement"=→"VDDIO_Voltage, V":dbl, "instrument handle out"=w381:refnum<k15>)  [unwired: 6 in, 1 out]
        n218 = call <instrlib>:"niDCPower Measure.vi"("measurement type"=w378, "channel name"="0", "instrument handle"=w381) -> ("measurement"=w382:dbl, "instrument handle out"=w371:refnum<k15>)  [unwired: 6 in, 1 out]
        n219 = Multiply(x=w382, y=1000.0) -> (x*y=→"VDDIO_Current, mA":dbl)
      }
    }
    n220 = call <instrlib>:"niDCPower Configure Output Enabled.vi"("output enabled"="output enabled", "channel name"="0", "instrument handle"=w341) -> ("instrument handle out"=w353:refnum<k15>)  [unwired: 7 in, 1 out]
    n221 = call <instrlib>:"niDCPower Measure.vi"("measurement type"=w346, "channel name"="0", "instrument handle"=w353) -> ("measurement"=→"VAA_Voltage, V":dbl, "instrument handle out"=w351:refnum<k15>)  [unwired: 6 in, 1 out]
    n222 = call <instrlib>:"niDCPower Measure.vi"("measurement type"=w345, "channel name"="0", "instrument handle"=w351) -> ("measurement"=w347:dbl, "instrument handle out"=w342:refnum<k15>)  [unwired: 6 in, 1 out]
    n223 = Multiply(x=w347, y=1000.0) -> (x*y=→"VAA_Current, mA":dbl)
    n224 = local read "stop"() -> (w356:bool)
    n225 = Wait (ms)(milliseconds to wait=u32 1) -> ()  [unwired: 1 out]
  }
  n226 = while {
    shift-right: [w384] -> _
    shift-left: FALSE -> [w387]
    tunnel: w3 -> [_]
    stop <- w388 stop-if-true
    # "Инициализация"
    n227 = local read "output enabled"() -> (w384:bool)
    n228 = Greater?(x=w384, y=w387) -> (0:w386:bool)
    n229 = case shown="True" w386 {
      frame False {
      }
      frame True {
        n230 = stacked-sequence {
          frame #0 {
            n231 = local write "/RESET"(FALSE ("RESET")) -> ()
            n232 = Wait (ms)(milliseconds to wait=u32 50) -> ()  [unwired: 1 out]
          }
          frame #1 {
            n233 = local write "/RESET"(TRUE ("RESET")) -> ()
            n234 = Wait (ms)(milliseconds to wait=u32 20) -> ()  [unwired: 1 out]
          }
          frame #2 {
            n235 = flat-sequence {
              frame #0 {
                n236 = local write "Comand"(T1."250x250" ("Comand")) -> ()
              }
              frame #1 {
                n237 = local write "Comand"(TRUE) -> ()
                n238 = Wait (ms)(milliseconds to wait=u32 20) -> ()  [unwired: 1 out]
              }
            }
          }
          frame #3 {
            n239 = flat-sequence {
              frame #0 {
                n240 = local write "Comand"(T1."From Controls" ("Comand")) -> ()
              }
              frame #1 {
                n241 = local write "Comand"(TRUE) -> ()
                n242 = Wait (ms)(milliseconds to wait=u32 20) -> ()  [unwired: 1 out]
              }
            }
          }
        }
      }
    }
    n243 = local read "stop"() -> (w388:bool)
    n244 = Wait (ms)(milliseconds to wait=u32 1) -> ()  [unwired: 1 out]
  }
  n245 = while {
    tunnel: w3 -> [w458]
    tunnel: [w458] -> w12
    shift-right: [w440] -> _
    shift-left: FALSE -> [w459]
    tunnel: w5 -> [_]
    shift-right: [w421] -> _
    shift-left: TRUE -> [w422]
    stop <- w420 stop-if-true
    # "Массивы переворачиваются!!!!!!"
    n246 = local read "Device"() -> (w417:u8)
    n247 = local read "ArrayLow"() -> (w434:u64)
    n248 = local read "ArrayUp"() -> (w433:u64)
    n249 = Increment(x=w417) -> (x+1=w416:u8)
    n250 = local read "Reg"() -> (w415:u8)
    n251 = xnode "Read/Write Control"("FPGA VI Reference In"=w458, "I2C_Write"="I2C_Write", "Read2"="Read2", "Read1"="Read1", "Device_Read"=w416, "Reg"=w415, "Device_Write"=w417, "91"="91", "100_Sclk_divider"="100_Sclk_divider", "75_Stop"="75_Stop", "53"="53", "35"="35", "17"="17", "71"="71", "54"="54", "36"="36", "18"="18", "72"="72", "50_Rise/Fall divider"="50_Rise/Fall divider", "0_WE divider"="0_WE divider", "DataUp"=w433, "DataLow"=w434, "I2C_Request"="I2C_Request", "FALSE_LV"="FALSE_LV", "FALSE_PIXCLK"="FALSE_PIXCLK", "TRUE_FV"="TRUE_FV", "Остановите"="stop", "Читай_Линию"=w422, "1_EXTCLK_divider"="1_EXTCLK_divider", "String_number"="String_number", "55"="55", "56"="56", "75"="75", "73"="73", "55"="55", "RESET"="/RESET", "57"="57") -> ("FPGA VI Reference Out"=w457:refnum<k20>, "Линия_готова_на_все"=w440:bool, "ACK"=w429:bool[], "String_counter"=→"String_counter":i16, "READ_Number"=w401:u64)  [unwired: 2 in, 3 out]
    "number" <- w401
    n252 = Number To Boolean Array(number=w401) -> (Boolean array=w402:bool[])
    n253 = Greater?(x=w440, y=w459) -> (0:w430:bool)
    n254 = Boolean Array To Number(Boolean array=w429) -> (number=→"ACK":u8)
    n255 = case shown="True" w430 {
      tunnel: w457 -> [_ w487]
      tunnel: [TRUE FALSE ("Читай_Линию")] -> w421
      frame False {
      }
      frame True {
        # "Чтение из FIFO данных (картинка)"
        n256 = xnode "Invoke Method"("FPGA VI Reference In"=w487, "Number of Elements"=u32 0, "Timeout (ms)"=0) -> ("FPGA VI Reference Out"=w492:refnum<k20>, "error out"=w491:errorcluster, "Elements Remaining"=w483:u32)  [unwired: 1 in, 1 out]
        "Сколько вначале" <- w483
        n257 = xnode "Invoke Method"("FPGA VI Reference In"=w492, "error in"=w491, "Number of Elements"=w483, "Timeout (ms)"=0) -> ("FPGA VI Reference Out"=w484:refnum<k20>, "Data"=→"Data":u8[])  [unwired: 2 out]
        n258 = Not(x=TRUE) -> (.not. x?=w485:bool)
        n259 = xnode "Read/Write Control"("FPGA VI Reference In"=w484, "Линия_ прочтена"=w485) -> ()  [unwired: 1 in, 2 out]
        "Ready" <- TRUE ("Ready")
      }
    }
    n260 = Split 1D Array(array=w402, index=6) -> (second subarray=w413:bool[])  [unwired: 1 out]
    n261 = Split 1D Array(array=w413, index=16) -> (first subarray=w411:bool[], second subarray=w409:bool[])
    n262 = for {
      tunnel: w411 -> [w470] mode=indexing
      shift-right: [w469] -> w410
      shift-left: bool[] [] -> [w468]
      tunnel: w409 -> [w462] mode=indexing
      shift-right: [w461] -> w408
      shift-left: bool[] [] -> [w460]
      i -> [w465]
      n263 = Quotient & Remainder(x=w465, y=2) -> (x-y*floor(x/y)=w467:i32)  [unwired: 1 out]
      n264 = Equal?(x=w467, y=1) -> (x = y?=w466:bool)
      n265 = case shown="True" w466 {
        tunnel: w470 -> [_ w478]
        tunnel: [w472 w477] -> w469
        tunnel: w468 -> [w472 w476]
        tunnel: w462 -> [_ w475]
        tunnel: [w471 w474] -> w461
        tunnel: w460 -> [w471 w473]
        frame False {
        }
        frame True {
          n266 = Build Array (concatenate)(w478, w476) -> (w477:bool[])
          n267 = Build Array (concatenate)(w475, w473) -> (w474:bool[])
        }
      }
    }
    n268 = Boolean Array To Number(Boolean array=w410) -> (number=w400:u8)
    "Read_Up" <- w400
    n269 = Boolean Array To Number(Boolean array=w408) -> (number=w399:u8)
    "Read_Low" <- w399
    n270 = Join Numbers(hi=w400, lo=w399) -> ((hi.lo)=→"Data_Read":u16)
    n271 = local read "stop"() -> (w420:bool)
    n272 = Wait (ms)(milliseconds to wait=u32 1) -> ()  [unwired: 1 out]
  }
  n273 = flat-sequence {
    tunnel: w9 -> [w495]
    frame #0 {
      n274 = call <instrlib>:"niDCPower Configure Output Enabled.vi"("output enabled"=FALSE, "instrument handle"=w495) -> ("instrument handle out"=w493:refnum<k15>)  [unwired: 8 in, 1 out]
      n275 = call <instrlib>:"niDCPower Close.vi"("instrument handle"=w493) -> ()  [unwired: 10 in, 1 out]
    }
  }
  n276 = flat-sequence {
    tunnel: w1 -> [w498]
    frame #0 {
      n277 = call <instrlib>:"niDCPower Configure Output Enabled.vi"("output enabled"=FALSE, "instrument handle"=w498) -> ("instrument handle out"=w496:refnum<k15>)  [unwired: 8 in, 1 out]
      n278 = call <instrlib>:"niDCPower Close.vi"("instrument handle"=w496) -> ()  [unwired: 10 in, 1 out]
    }
  }
  n279 = xnode "Close FPGA VI Reference"("FPGA VI Reference In"=w12) -> ()  [unwired: 1 in, 1 out]
